vi "ws_runtest initialize fields.vi"(4 "Process SPARTAN SN (F)":bool, 6 "User/Station":T8, 7 "POST (empty)":T6, 8 "error in (no error)":errorcluster, 9 "ProcessNextItem? (f)":bool, 10 "Test Sequence ID":string, 11 "Connection Refnum":T7) -> (0 "error out":errorcluster, 1 "Fields / Results":T5, 2 "dup Test Sequence ID":string, 3 "Connection Refnum":T7, 5 "POST out":T6)   [LabVIEW 2011]
uses:
  <vilib>/addons/internet/utils/keyedarr.llb/Keyed Array.ctl
  SI.LIB/ODBC/SQL Controls/Connection Refnum.ctl
  runtest User - Station.ctl
  server/database/Stations/Instruments/Instrument Record.ctl
  server/database/Stations/Step Associations/Step Association Record.ctl
  server/database/Fields/Field Record.ctl
  server/database/Fields/Field DataTypes.ctl
  server/database/Fields/Field NextItem.ctl
  tests/Test Output.ctl
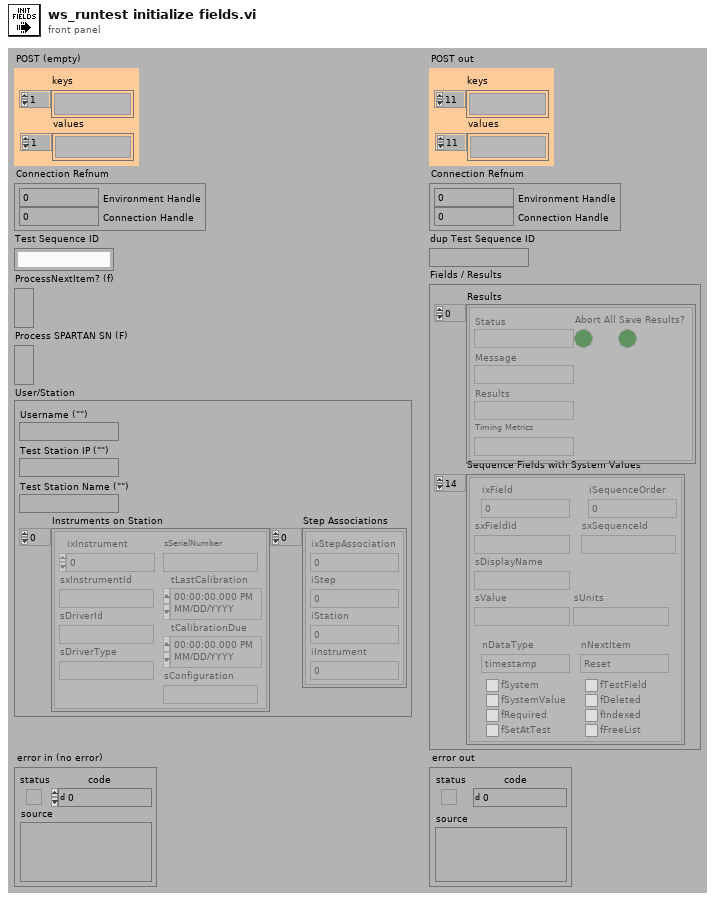
[diagram p1: front panel]
types:
  T1 = typedef "Field Record.ctl" = cluster{"ixField":i32, "iSequenceOrder":i32, "sxFieldId":string, "sxSequenceId":string, "sDisplayName":string, "sValue":string, "sUnits":string, "nDataType":T2, "nNextItem":T3, "fSystem":bool, "fSystemValue":bool, "fRequired":bool, "fSetAtTest":bool, "fTestField":bool, "fDeleted":bool, "fIndexed":bool, "fFreeList":bool}
  T2 = typedef "Field DataTypes.ctl" = enum32{"text", "numeric", "list", "timestamp", "boolean"}
  T3 = typedef "Field NextItem.ctl" = enum32{"Reset", "Retain", "Auto-Increment"}
  T4 = typedef "Test Output.ctl" = cluster{"Status":string, "Message":string, "Results":string, "Abort All":bool, "Save Results?":bool, "Timing Metrics":string}
  T5 = cluster{"Sequence Fields with System Values":T1[], "Results":T4[]}
  T6 = typedef "Keyed Array.ctl" = cluster{"keys":string[], "values":string[]}
  T7 = typedef "Connection Refnum.ctl" = cluster{"Environment Handle":i32, "Connection Handle":i32}
  T8 = typedef "runtest User - Station.ctl" = cluster{"Username (\"\")":string, "Test Station IP (\"\")":string, "Test Station Name (\"\")":string, "Instruments on Station":T9[], "Step Associations":T10[]}
  T9 = typedef "Instrument Record.ctl" = cluster{"ixInstrument":i32, "sxInstrumentId":string, "sDriverId":string, "sDriverType":string, "sSerialNumber":string, "tLastCalibration":timestamp, "tCalibrationDue":timestamp, "sConfiguration":string}
  T10 = typedef "Step Association Record.ctl" = cluster{"ixStepAssociation":i32, "iStep":i32, "iStation":i32, "iInstrument":i32}
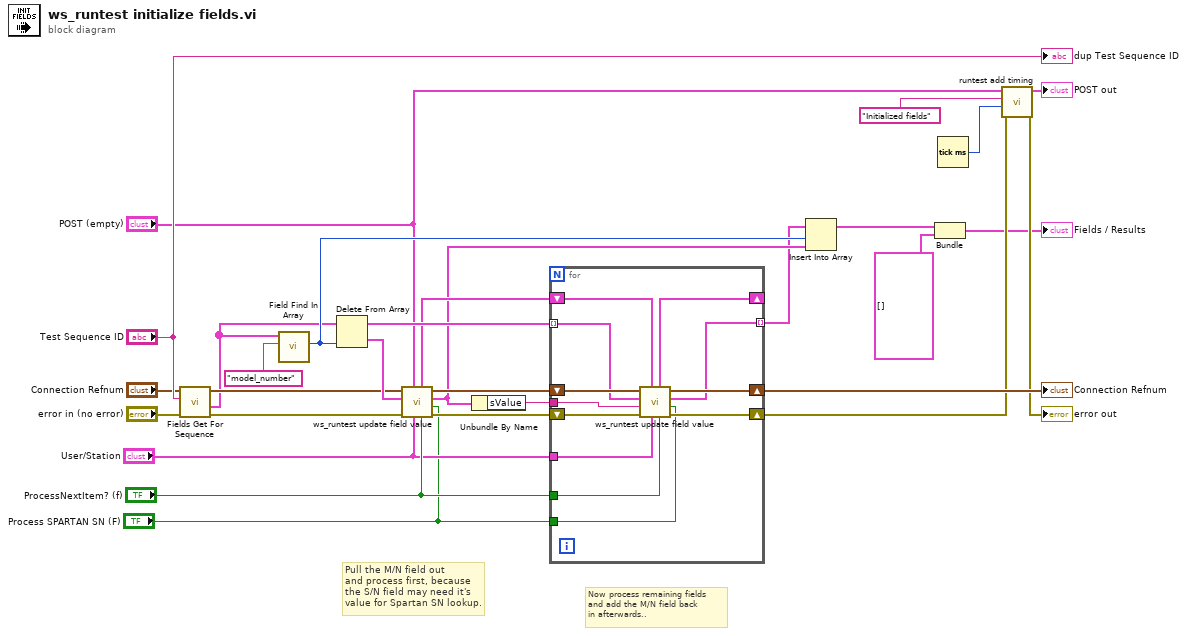
[diagram p0: block diagram]
diagram:
  # "Now process remaining fields\nand add the M/N field back\nin afterwards.."
  # "Pull the M/N field out\nand process first, because\nthe S/N field may need it's\nvalue for Spartan SN lookup."
  n1 = call "Fields Get For Sequence.vi"("error in (no error)"="error in (no error)", "sxSequenceId (\"\")"="Test Sequence ID", "Connection Refnum"="Connection Refnum") -> ("error out"=w3:errorcluster, "Current Sequence Fields"=w4:T1[], "Connection Refnum"=w5:T7)  [unwired: 6 out]
  n2 = call "Field Find In Array.vi"("FieldID or Display Name(\"\")"="model_number", "Field Array"=w4) -> ("Index"=w28:i32)  [unwired: 1 in, 8 out]
  n3 = Delete From Array(array=w4, index=w28) -> (deleted portion=w20:T1, array with subset deleted=w27:T1[])  [unwired: 1 in]
  n4 = call "ws_runtest update field value.vi"("Process SPARTAN SN (F)"="Process SPARTAN SN (F)", "ProcessNextItem? (f)"="ProcessNextItem? (f)", "User/Station"="User/Station", "POST (empty)"="POST (empty)", "error in (no error)"=w3, "Field"=w20, "Connection Refnum"=w5) -> ("error out"=w26:errorcluster, "updated Field"=w23:T1, "Connection Refnum"=w25:T7, "remaining POST"=w24:T6)  [unwired: 1 in]
  n5 = Unbundle By Name(w23) -> ("sValue"=w22:string)
  n6 = for {
    tunnel: w27 -> [w32] mode=indexing
    shift-right: [w37] -> _
    shift-left: w24 -> [w38]
    shift-right: [w39] -> w13
    shift-left: w26 -> [w40]
    shift-right: [w35] -> w19
    shift-left: w25 -> [w41]
    tunnel: w22 -> [w36]
    tunnel: [w34] -> w21 mode=indexing
    tunnel: "User/Station" -> [w33]
    tunnel: "ProcessNextItem? (f)" -> [w31]
    tunnel: "Process SPARTAN SN (F)" -> [w30]
    n7 = call "ws_runtest update field value.vi"("Process SPARTAN SN (F)"=w30, "ProcessNextItem? (f)"=w31, "User/Station"=w33, "POST (empty)"=w38, "error in (no error)"=w40, "Model Number (\"\")"=w36, "Field"=w32, "Connection Refnum"=w41) -> ("error out"=w39:errorcluster, "updated Field"=w34:T1, "Connection Refnum"=w35:T7, "remaining POST"=w37:T6)
  }
  "Connection Refnum" <- w19
  n8 = Insert Into Array(array=w21, index=w28, new element=w23) -> (w11:T1[])
  n9 = Bundle(w11, "Test Step Outputs"=T4[] []) -> (→"Fields / Results":cluster{T1[], "Test Step Outputs":T4[]})  [unwired: 1 out]
  n10 = Tick Count (ms)() -> (millisecond timer value=w14:u32)
  n11 = call "runtest add timing.vi"("error in (no error)"=w13, "Start Tick, ms (0)"=w14, "Function (\"\")"="Initialized fields", "POST (empty)"="POST (empty)") -> ("error out"=→"error out":errorcluster, "POST out"=→"POST out":T6)  [unwired: 6 out]
  "dup Test Sequence ID" <- "Test Sequence ID"
